vi "LM Two T-Connected Asymmetric Gaussians and gradient.vi"(3 "output control":T1, 4 "data":variant, 5 "X":dbl[](array[numeric]), 6 "a":dbl[](array[numeric])) -> (0 "error out":errorcluster, 1 "f'(X,a)":dbl[][](array[numeric]), 2 "f(X,a)":dbl[](array[numeric]))   [LabVIEW 2019]
doc: "This template is the starting point for creating a model function to be passed to the Nonlinear Curve Fit.vi."
uses:
  <vilib>/gmath/NumericalOptimization/LM_output select.ctl
  D-Only Fixed Parameters.ctl
  <vilib>/gmath/NI_Gmath.lvlib
panel:
  # "Parameters:\n\namplitude 1: A1\ncenter 1: t1\nSDV 1-: s1p\nSDV 1+: s1m \n\nAmplitude 2: A2\ncenter 2: t2\nSDV 2-: s2m\nSDV 2+: s2p\n\nBridge Amplitude: A3 (or b)\nBridge Slope: a"
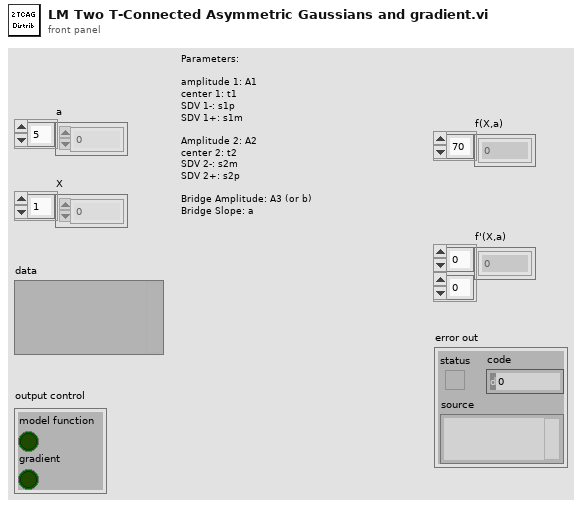
[diagram p1: front panel]
types:
  T1 = typedef "NI_Gmath.lvlib/LM_output select.ctl" = cluster{"model function":bool, "gradient":bool}
  T2 = typedef "D-Only Fixed Parameters.ctl" = cluster{"Fix D-only Peak Location":bool, "Peak Location":dbl, "Fix D-only Peak FWHM":bool, "Peak FWHM":dbl}
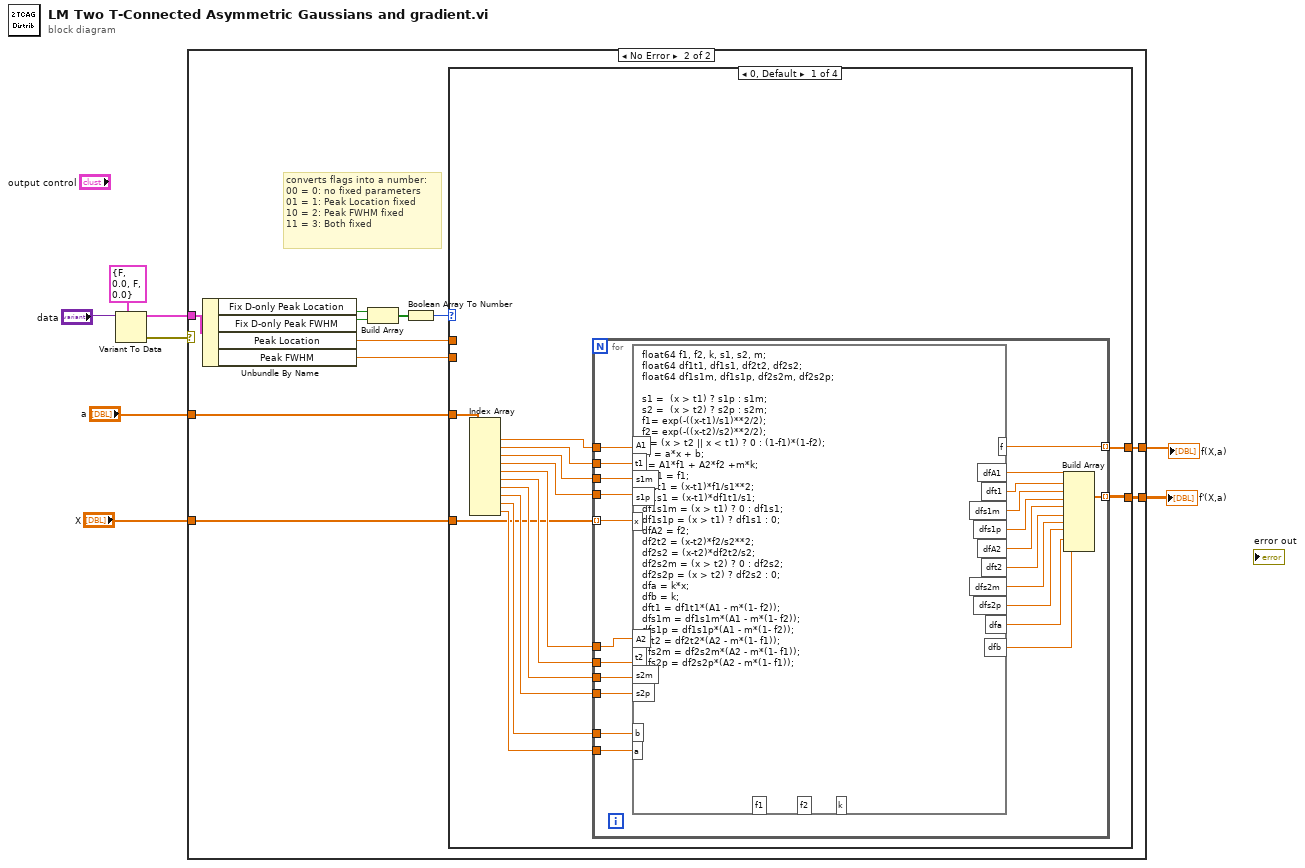
[diagram p0: block diagram]
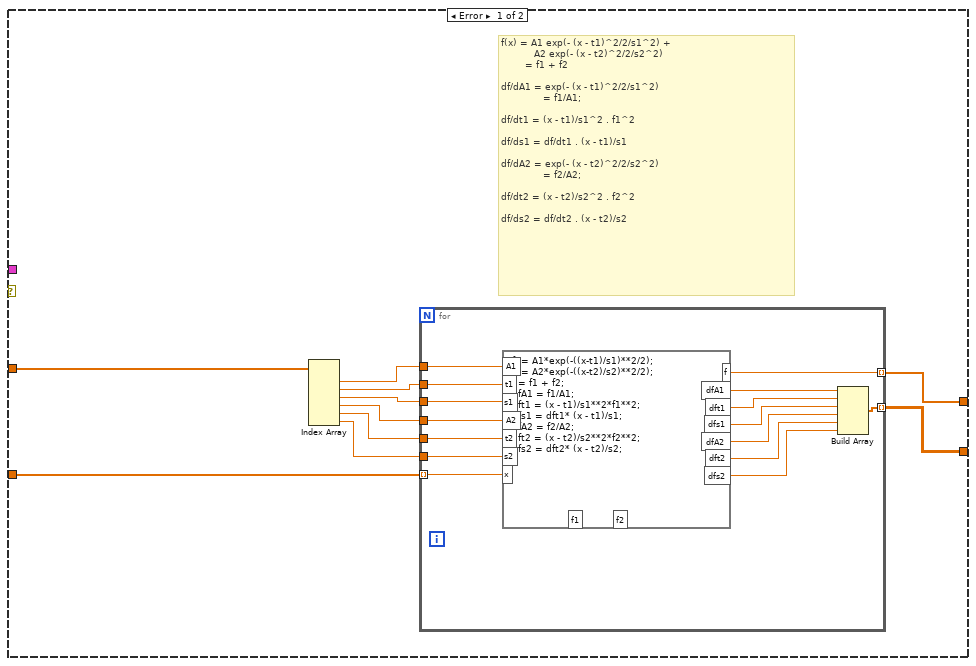
[diagram p2: hidden frame]
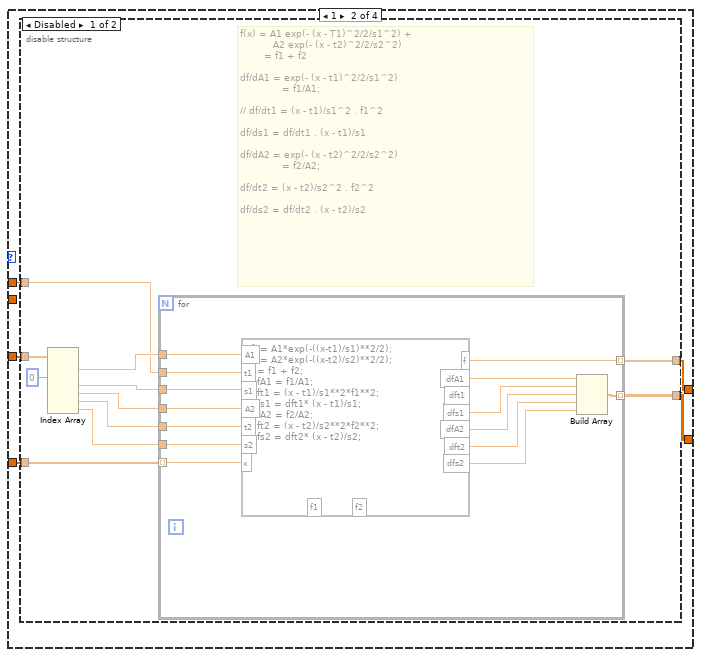
[diagram p3: hidden frame]
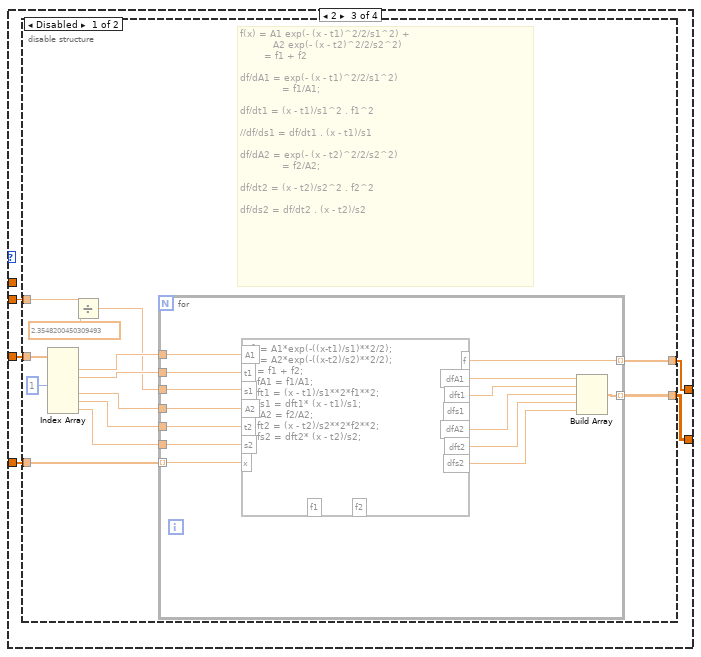
[diagram p5: hidden frame]
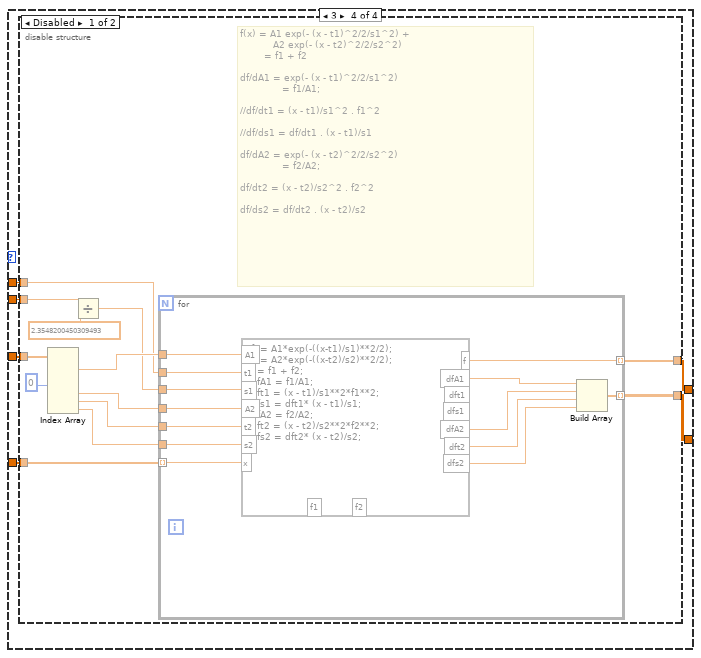
[diagram p7: hidden frame]
diagram:
  n1 = Variant To Data(type=T2 {"Fix D-only Peak Location"=FALSE, "Peak Location"=0.0, "Fix D-only Peak FWHM"=FALSE, "Peak FWHM"=0.0} ("Fixed Parameters"), Variant="data") -> (data=w1:T2, error out=w2:errorcluster)  [unwired: 1 in]
  n2 = case shown="No Error" w2 {
    tunnel: "a" -> [w18 w44]
    tunnel: "X" -> [w17 w43]
    tunnel: [w16 w42] -> w6
    tunnel: [w15 w41] -> w5
    tunnel: w1 -> [_ w40]
    frame Error {
      # "f(x) = A1 exp(- (x - t1)^2/2/s1^2) +\n           A2 exp(- (x - t2)^2/2/s2^2)\n        = f1 + f2\n\ndf/dA1 = exp(- (x - t1)^2/2/s1^2)\n              = f1/A1;\n\ndf/dt1 = (x - t1)/s1^2 . f1^2\n\ndf/ds1 = df/dt1 . (x - t1)/s1                     \n\ndf/dA2 = exp(- (x - t2)^2/2/s2^2)\n              = f2/A2;\n\ndf/dt2 = (x - t2)/s2^2 . f2^2\n\ndf/ds2 = df/dt2 . (x - t2)/s2"
      n3 = Index Array(array=w18) -> (element #1=w14:dbl, element #2=w13:dbl, element #3=w12:dbl, element #4=w11:dbl, element #5=w10:dbl, element #6=w9:dbl)  [unwired: 6 in]
      n4 = for {
        tunnel: w17 -> [w33] mode=indexing
        tunnel: [w31] -> w16 mode=indexing
        tunnel: [w30] -> w15 mode=indexing
        tunnel: w14 -> [w29]
        tunnel: w13 -> [w28]
        tunnel: w12 -> [w27]
        tunnel: w11 -> [w26]
        tunnel: w10 -> [w25]
        tunnel: w9 -> [w24]
        n5 = formula code="f1= A1*exp(-((x-t1)/s1)**2/2);\nf2= A2*exp(-((x-t2)/s2)**2/2);\nf = f1 + f2;\ndfA1 = f1/A1;\ndft1 = (x - t1)/s1**2*f1**2;\ndfs1 = dft1* (x - t1)/s1;\ndfA2 = f2/A2;\ndft2 = (x - t2)/s2**2*f2**2;\ndfs2 = dft2* (x - t2)/s2;"("A1"=w29, "t1"=w28, "s1"=w27, "x"=w33, "A2"=w26, "t2"=w25, "s2"=w24) -> ("f"=w31:dbl, "dfA1"=w32:dbl, "dft1"=w23:dbl, "dfs1"=w22:dbl, "dfA2"=w21:dbl, "dft2"=w20:dbl, "dfs2"=w19:dbl)  [unwired: 2 out]
        n6 = Build Array(w32, w23, w22, w21, w20, w19) -> (w30:dbl[])
      }
    }
    frame No Error {
      # "converts flags into a number:\n00 = 0: no fixed parameters\n01 = 1: Peak Location fixed\n10 = 2: Peak FWHM fixed\n11 = 3: Both fixed"
      n7 = Unbundle By Name(w40) -> ("Fix D-only Peak Location"=w39:bool, "Fix D-only Peak FWHM"=w38:bool, "Peak Location"=w35:dbl, "Peak FWHM"=w34:dbl)
      n8 = Build Array(w39, w38) -> (w37:bool[])
      n9 = Boolean Array To Number(Boolean array=w37) -> (number=w36:u32)
      n10 = case shown="0, Default" w36 {
        tunnel: w44 -> [w48 w86 w116 w149]
        tunnel: w43 -> [w47 w85 w115 w148]
        tunnel: [w46 w84 w114 w147] -> w42
        tunnel: [w45 w83 w113 w146] -> w41
        tunnel: w35 -> [_ w82 _ w144]
        tunnel: w34 -> [_ _ w112 w145]
        frame 0, Default {
          n11 = Index Array(array=w48) -> (element #1=w49:dbl, element #2=w50:dbl, element #3=w51:dbl, element #4=w52:dbl, element #5=w53:dbl, element #6=w54:dbl, element #7=w55:dbl, element #8=w56:dbl, element #9=w57:dbl, element #10=w58:dbl)  [unwired: 10 in]
          n12 = for {
            tunnel: w49 -> [w73]
            tunnel: w50 -> [w74]
            tunnel: w51 -> [w75]
            tunnel: w52 -> [w76]
            tunnel: w47 -> [w72] mode=indexing
            tunnel: w53 -> [w77]
            tunnel: w54 -> [w78]
            tunnel: w55 -> [w79]
            tunnel: w56 -> [w80]
            tunnel: w57 -> [w81]
            tunnel: [w71] -> w46 mode=indexing
            tunnel: [w61] -> w45 mode=indexing
            tunnel: w58 -> [w60]
            n13 = formula code="float64 f1, f2, k, s1, s2, m;\nfloat64 df1t1, df1s1, df2t2, df2s2;\nfloat64 df1s1m, df1s1p, df2s2m, df2s2p;\n\ns1 =  (x > t1) ? s1p : s1m;\ns2 =  (x > t2) ? s2p : s2m;\nf1= exp(-((x-t1)/s1)**2/2);\nf2= exp(-((x-t2)/s2)**2/2);\nk = (x > t2 || x < t1) ? 0 : (1-f1)*(1-f2);\nm = a*x + b;\nf = A1*f1 + A2*f2 +m*k;\ndfA1 = f1;\ndf1t1 = (x-t1)*f1/s1**2;\ndf1s1 = (x-t1)*df1t1/s1;\ndf1s1m = (x > t1) ? 0 : df1s1;\ndf1s1p = (x > t1) ? df1s1 : 0;\ndfA2 = f2;\ndf2t2 = (x-t2)*f2/s2**2;\ndf2s2 = (x-t2)*df2t2/s2;\ndf2s2m = (x > t2) ? 0 : df2s2;\ndf2s2p = (x > t2) ? df2s2 : 0;\ndfa = k*x;\ndfb = k;\ndft1 = df1t1*(A1 - m*(1- f2));\ndfs1m = df1s1m*(A1 - m*(1- f2));\ndfs1p = df1s1p*(A1 - m*(1- f2));\ndft2 = df2t2*(A2 - m*(1- f1));\ndfs2m = df2s2m*(A2 - m*(1- f1));\ndfs2p = df2s2p*(A2 - m*(1- f1));"("A1"=w73, "t1"=w74, "s1m"=w75, "x"=w72, "A2"=w77, "t2"=w78, "s2m"=w79, "b"=w81, "s1p"=w76, "s2p"=w80, "a"=w60) -> ("f"=w71:dbl, "dfA1"=w70:dbl, "dft1"=w69:dbl, "dfs1m"=w68:dbl, "dfA2"=w66:dbl, "dft2"=w65:dbl, "dfs2m"=w64:dbl, "dfa"=w62:dbl, "dfs1p"=w67:dbl, "dfs2p"=w63:dbl, "dfb"=w59:dbl)  [unwired: 3 out]
            n14 = Build Array(w70, w69, w68, w67, w66, w65, w64, w63, w62, w59) -> (w61:dbl[])
          }
        }
        frame 1 {
          n15 = disable-structure shown="Disabled" {
            disable-tunnel: w86 -> [w97 _]
            disable-tunnel: w85 -> [w96 _]
            disable-tunnel: [w95 _] -> w84
            disable-tunnel: [w94 _] -> w83
            disable-tunnel: w82 -> [w88 _]
            frame Disabled {
              # "f(x) = A1 exp(- (x - T1)^2/2/s1^2) +\n           A2 exp(- (x - t2)^2/2/s2^2)\n        = f1 + f2\n\ndf/dA1 = exp(- (x - t1)^2/2/s1^2)\n              = f1/A1;\n\n// df/dt1 = (x - t1)/s1^2 . f1^2\n\ndf/ds1 = df/dt1 . (x - t1)/s1                     \n\ndf/dA2 = exp(- (x - t2)^2/2/s2^2)\n              = f2/A2;\n\ndf/dt2 = (x - t2)/s2^2 . f2^2\n\ndf/ds2 = df/dt2 . (x - t2)/s2"
              n16 = Index Array(array=w97, index #2=0 ("index")) -> (element #1=w93:dbl, element #3=w92:dbl, element #4=w91:dbl, element #5=w90:dbl, element #6=w89:dbl)  [unwired: 5 in, 1 out]
              n17 = for {
                tunnel: w96 -> [w111] mode=indexing
                tunnel: [w109] -> w95 mode=indexing
                tunnel: [w108] -> w94 mode=indexing
                tunnel: w93 -> [w107]
                tunnel: w88 -> [w106]
                tunnel: w92 -> [w105]
                tunnel: w91 -> [w104]
                tunnel: w90 -> [w103]
                tunnel: w89 -> [w102]
                n18 = formula code="f1= A1*exp(-((x-t1)/s1)**2/2);\nf2= A2*exp(-((x-t2)/s2)**2/2);\nf = f1 + f2;\ndfA1 = f1/A1;\ndft1 = (x - t1)/s1**2*f1**2;\ndfs1 = dft1* (x - t1)/s1;\ndfA2 = f2/A2;\ndft2 = (x - t2)/s2**2*f2**2;\ndfs2 = dft2* (x - t2)/s2;"("A1"=w107, "t1"=w106, "s1"=w105, "x"=w111, "A2"=w104, "t2"=w103, "s2"=w102) -> ("f"=w109:dbl, "dfA1"=w110:dbl, "dfs1"=w101:dbl, "dfA2"=w100:dbl, "dft2"=w99:dbl, "dfs2"=w98:dbl)  [unwired: 3 out]
                n19 = Build Array(w110, w101, w100, w99, w98) -> (w108:dbl[])
              }
            }
            frame Enabled {
            }
          }
        }
        frame 2 {
          n20 = disable-structure shown="Disabled" {
            disable-tunnel: w116 -> [w129 _]
            disable-tunnel: w115 -> [w128 _]
            disable-tunnel: [w127 _] -> w114
            disable-tunnel: [w126 _] -> w113
            disable-tunnel: w112 -> [w120 _]
            frame Disabled {
              # "f(x) = A1 exp(- (x - t1)^2/2/s1^2) +\n           A2 exp(- (x - t2)^2/2/s2^2)\n        = f1 + f2\n\ndf/dA1 = exp(- (x - t1)^2/2/s1^2)\n              = f1/A1;\n\ndf/dt1 = (x - t1)/s1^2 . f1^2\n\n//df/ds1 = df/dt1 . (x - t1)/s1                     \n\ndf/dA2 = exp(- (x - t2)^2/2/s2^2)\n              = f2/A2;\n\ndf/dt2 = (x - t2)/s2^2 . f2^2\n\ndf/ds2 = df/dt2 . (x - t2)/s2"
              n21 = Index Array(array=w129, index #3=1 ("index")) -> (element #1=w125:dbl, element #2=w124:dbl, element #4=w123:dbl, element #5=w122:dbl, element #6=w121:dbl)  [unwired: 5 in, 1 out]
              n22 = Divide(x=w120, y=2.3548200450309493) -> (x/y=w118:dbl)
              n23 = for {
                tunnel: w128 -> [w143] mode=indexing
                tunnel: [w141] -> w127 mode=indexing
                tunnel: [w140] -> w126 mode=indexing
                tunnel: w125 -> [w139]
                tunnel: w124 -> [w138]
                tunnel: w118 -> [w137]
                tunnel: w123 -> [w136]
                tunnel: w122 -> [w135]
                tunnel: w121 -> [w134]
                n24 = formula code="f1= A1*exp(-((x-t1)/s1)**2/2);\nf2= A2*exp(-((x-t2)/s2)**2/2);\nf = f1 + f2;\ndfA1 = f1/A1;\ndft1 = (x - t1)/s1**2*f1**2;\ndfs1 = dft1* (x - t1)/s1;\ndfA2 = f2/A2;\ndft2 = (x - t2)/s2**2*f2**2;\ndfs2 = dft2* (x - t2)/s2;"("A1"=w139, "t1"=w138, "s1"=w137, "x"=w143, "A2"=w136, "t2"=w135, "s2"=w134) -> ("f"=w141:dbl, "dfA1"=w142:dbl, "dft1"=w133:dbl, "dfA2"=w132:dbl, "dft2"=w131:dbl, "dfs2"=w130:dbl)  [unwired: 3 out]
                n25 = Build Array(w142, w133, w132, w131, w130) -> (w140:dbl[])
              }
            }
            frame Enabled {
            }
          }
        }
        frame 3 {
          n26 = disable-structure shown="Disabled" {
            disable-tunnel: w149 -> [w162 _]
            disable-tunnel: w148 -> [w161 _]
            disable-tunnel: [w160 _] -> w147
            disable-tunnel: [w159 _] -> w146
            disable-tunnel: w145 -> [w154 _]
            disable-tunnel: w144 -> [w151 _]
            frame Disabled {
              # "f(x) = A1 exp(- (x - t1)^2/2/s1^2) +\n           A2 exp(- (x - t2)^2/2/s2^2)\n        = f1 + f2\n\ndf/dA1 = exp(- (x - t1)^2/2/s1^2)\n              = f1/A1;\n\n//df/dt1 = (x - t1)/s1^2 . f1^2\n\n//df/ds1 = df/dt1 . (x - t1)/s1                     \n\ndf/dA2 = exp(- (x - t2)^2/2/s2^2)\n              = f2/A2;\n\ndf/dt2 = (x - t2)/s2^2 . f2^2\n\ndf/ds2 = df/dt2 . (x - t2)/s2"
              n27 = Index Array(array=w162, index #3=0 ("index")) -> (element #1=w158:dbl, element #4=w157:dbl, element #5=w156:dbl, element #6=w155:dbl)  [unwired: 5 in, 2 out]
              n28 = Divide(x=w154, y=2.3548200450309493) -> (x/y=w152:dbl)
              n29 = for {
                tunnel: w161 -> [w175] mode=indexing
                tunnel: [w173] -> w160 mode=indexing
                tunnel: [w172] -> w159 mode=indexing
                tunnel: w158 -> [w171]
                tunnel: w151 -> [w170]
                tunnel: w152 -> [w169]
                tunnel: w157 -> [w168]
                tunnel: w156 -> [w167]
                tunnel: w155 -> [w166]
                n30 = formula code="f1= A1*exp(-((x-t1)/s1)**2/2);\nf2= A2*exp(-((x-t2)/s2)**2/2);\nf = f1 + f2;\ndfA1 = f1/A1;\ndft1 = (x - t1)/s1**2*f1**2;\ndfs1 = dft1* (x - t1)/s1;\ndfA2 = f2/A2;\ndft2 = (x - t2)/s2**2*f2**2;\ndfs2 = dft2* (x - t2)/s2;"("A1"=w171, "t1"=w170, "s1"=w169, "x"=w175, "A2"=w168, "t2"=w167, "s2"=w166) -> ("f"=w173:dbl, "dfA1"=w174:dbl, "dfA2"=w165:dbl, "dft2"=w164:dbl, "dfs2"=w163:dbl)  [unwired: 4 out]
                n31 = Build Array(w174, w165, w164, w163) -> (w172:dbl[])
              }
            }
            frame Enabled {
            }
          }
        }
      }
    }
  }
  "f(X,a)" <- w6
  "f'(X,a)" <- w5
